vi "Calculate Formation Energies -(old).vi"(4 "N Extrinsic Atoms":i32, 5 "Fermi (electron) energy (eV)":dbl=-2.0, 6 "# Extra Electrons":i32, 7 "Reference Elemental Bulk Energies":T3={"Energy of CdTe (eV/atom)"=-2.489625, "Energy of Cd (eV/atom)"=-0.9039318, "Energy of Te (eV/atom)"=-3.1404524}, 8 "N (Te,ideal - Te,defect)":i32, 9 "N (Cd,Ideal - Cd,Defect)":i32, 10 "Reference Pure Structure Energy":dbl=-358.247, 11 "Final Total Defect Energy (eV)":dbl=-2.48963) -> (2 "Formation Energy (Te-Rich)":dbl, 3 "Formation Energy (Cd-Rich)":dbl)   [LabVIEW 2010]
panel:
  in  "System Array":T1(array[cluster])
  in  "System Cluster":T2={"Final Total Defect Energy (eV)"=-2.48963, "Reference Pure Structure Energy"=-358.247, "N (Cd,Ideal - Cd,Defect)"=0, "N (Te,ideal - Te,defect)"=0, "# Extra Electrons"=0, "Fermi (electron) energy (eV)"=-2.0}
  out "EForm 2":dbl
  out "Ed2 2":dbl
  out "Deltau 2":dbl
  out "uCd 2":dbl
  in  "uTe 2":dbl
  in  "Energy of Extrinsic X (eV/atom)":dbl
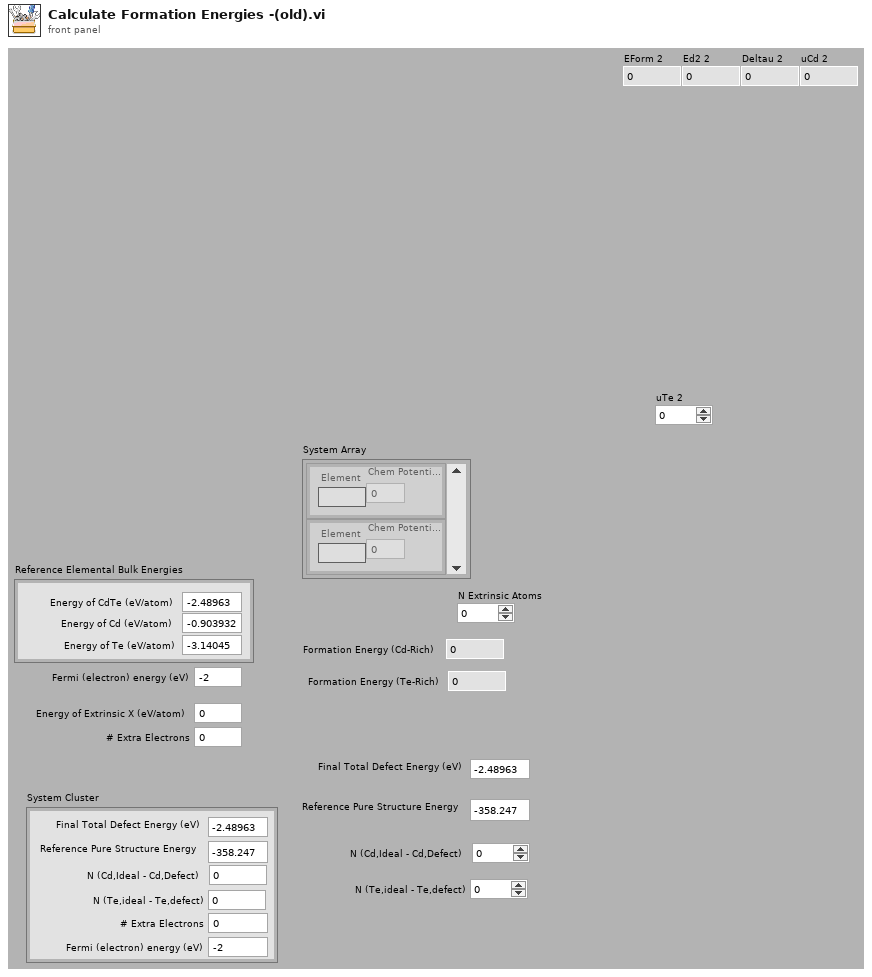
[diagram p1: front panel]
types:
  T1 = cluster{"Chem Potential (ev/atom)":dbl, "Element":string}[]
  T2 = cluster{"Final Total Defect Energy (eV)":dbl, "Reference Pure Structure Energy":dbl, "N (Cd,Ideal - Cd,Defect)":i32, "N (Te,ideal - Te,defect)":i32, "# Extra Electrons":i32, "Fermi (electron) energy (eV)":dbl}
  T3 = cluster{"Energy of CdTe (eV/atom)":dbl, "Energy of Cd (eV/atom)":dbl, "Energy of Te (eV/atom)":dbl}
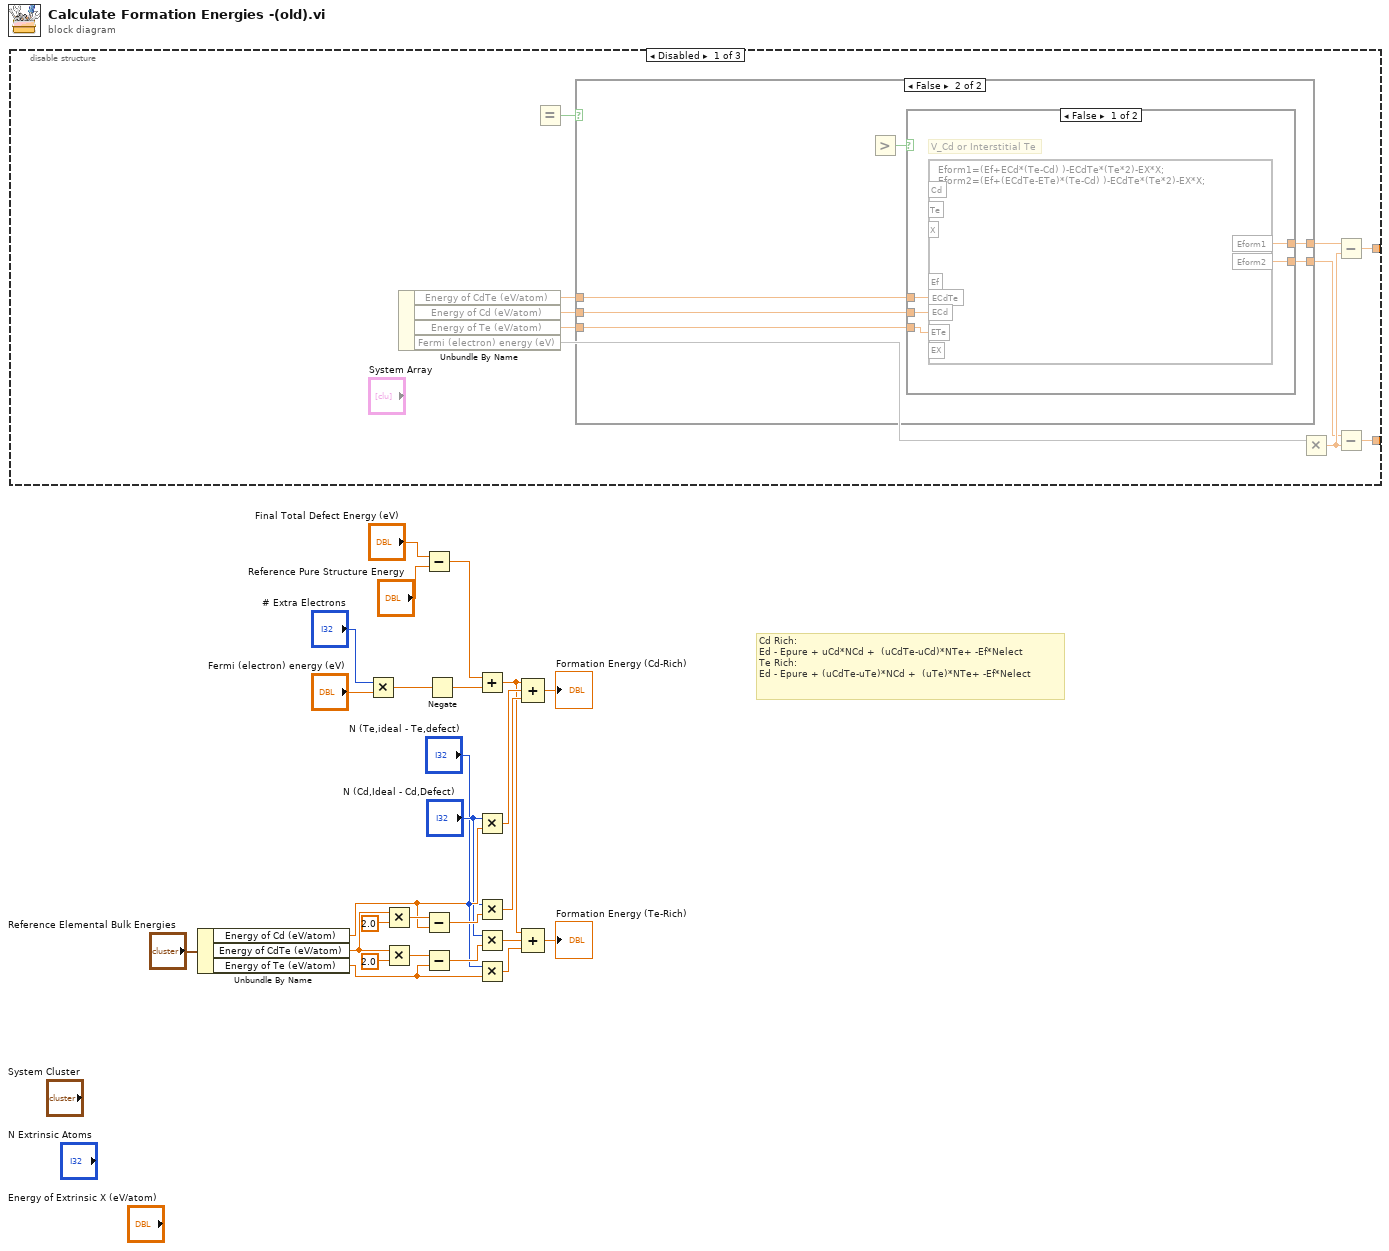
[diagram p0: block diagram]
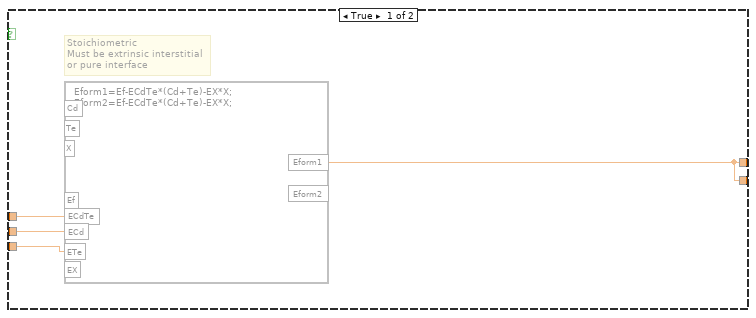
[diagram p2: hidden frame]
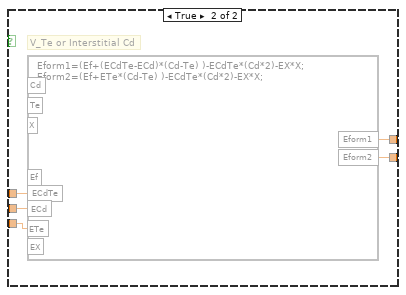
[diagram p3: hidden frame]
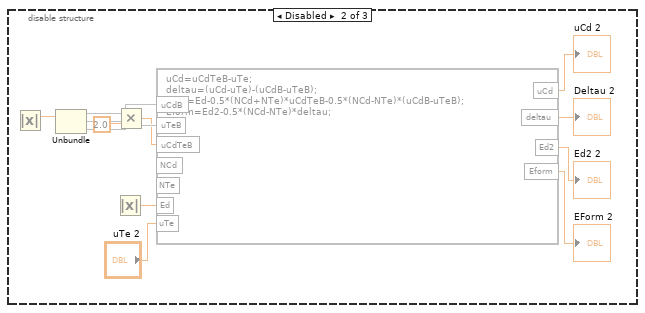
[diagram p4: hidden frame]
diagram:
  # "Cd Rich:\nEd - Epure + uCd*NCd +  (uCdTe-uCd)*NTe+ -Ef*Nelect\nTe Rich:\nEd - Epure + (uCdTe-uTe)*NCd +  (uTe)*NTe+ -Ef*Nelect"
  n1 = disable-structure shown="Disabled" {
    disable-tunnel: [w28 _ _] -> _
    disable-tunnel: [w27 _ _] -> _
    frame Disabled {
      n2 = Unbundle By Name() -> ("Energy of CdTe (eV/atom)"=w35:dbl, "Energy of Cd (eV/atom)"=w34:dbl, "Energy of Te (eV/atom)"=w33:dbl, "Fermi (electron) energy (eV)"=w32)  [unwired: 1 in]
      n3 = Equal?() -> (x = y?=w36:bool)  [unwired: 2 in]
      n4 = case shown="False" w36 {
        tunnel: w35 -> [w40 w46]
        tunnel: [w37 w42] -> w31
        tunnel: [w37 w41] -> w29
        tunnel: w34 -> [w39 w45]
        tunnel: w33 -> [w38 w44]
        frame True {
          # "Stoichiometric\nMust be extrinsic interstitial\nor pure interface"
          n5 = formula code="Eform1=Ef-ECdTe*(Cd+Te)-EX*X;\nEform2=Ef-ECdTe*(Cd+Te)-EX*X;"("ECdTe"=w40, "ECd"=w39, "ETe"=w38) -> ("Eform1"=w37:dbl)  [unwired: 5 in, 1 out]
        }
        frame False {
          n6 = Greater?() -> (0:w43:bool)  [unwired: 2 in]
          n7 = case shown="False" w43 {
            tunnel: w46 -> [w51 w56]
            tunnel: w45 -> [w50 w55]
            tunnel: w44 -> [w49 w54]
            tunnel: [w47 w52] -> w41
            tunnel: [w48 w53] -> w42
            frame False {
              # "V_Cd or Interstitial Te"
              n8 = formula code="Eform1=(Ef+ECd*(Te-Cd) )-ECdTe*(Te*2)-EX*X;\nEform2=(Ef+(ECdTe-ETe)*(Te-Cd) )-ECdTe*(Te*2)-EX*X;"("ECdTe"=w51, "ECd"=w50, "ETe"=w49) -> ("Eform1"=w48:dbl, "Eform2"=w47:dbl)  [unwired: 5 in]
            }
            frame True {
              # "V_Te or Interstitial Cd"
              n9 = formula code="Eform1=(Ef+(ECdTe-ECd)*(Cd-Te) )-ECdTe*(Cd*2)-EX*X;\nEform2=(Ef+ETe*(Cd-Te) )-ECdTe*(Cd*2)-EX*X;"("ECdTe"=w56, "ECd"=w55, "ETe"=w54) -> ("Eform1"=w53:dbl, "Eform2"=w52:dbl)  [unwired: 5 in]
            }
          }
        }
      }
      n10 = Multiply(x=w32) -> (x*y=w30:dbl)  [unwired: 1 in]
      n11 = Subtract(x=w31, y=w30) -> (x-y=w27:dbl)
      n12 = Subtract(x=w29, y=w30) -> (x-y=w28:dbl)
    }
    frame Disabled {
      n13 = Absolute Value() -> (abs(x)=w61:dbl)  [unwired: 1 in]
      n14 = Unbundle(w61) -> (w59, w68, w67)
      n15 = Absolute Value() -> (abs(x)=w60:dbl)  [unwired: 1 in]
      n16 = Multiply(x=w59, y=2.0) -> (x*y=w57:dbl)
      n17 = formula code="uCd=uCdTeB-uTe;\ndeltau=(uCd-uTe)-(uCdB-uTeB);\nEd2 =Ed-0.5*(NCd+NTe)*uCdTeB-0.5*(NCd-NTe)*(uCdB-uTeB);\nEform=Ed2-0.5*(NCd-NTe)*deltau;"("uCdB"=w68, "uTeB"=w67, "uCdTeB"=w57, "uTe"="uTe 2", "Ed"=w60) -> ("uCd"=→"uCd 2":dbl, "deltau"=→"Deltau 2":dbl, "Ed2"=→"Ed2 2":dbl, "Eform"=→"EForm 2":dbl)  [unwired: 2 in]
    }
    frame Enabled {
    }
  }
  n18 = Unbundle By Name("Reference Elemental Bulk Energies") -> ("Energy of Cd (eV/atom)"=w10:dbl, "Energy of CdTe (eV/atom)"=w11:dbl, "Energy of Te (eV/atom)"=w8:dbl)
  n19 = Multiply(x="# Extra Electrons", y="Fermi (electron) energy (eV)") -> (x*y=w5:dbl)
  n20 = Multiply(x=w11, y=2.0) -> (x*y=w12:dbl)
  n21 = Multiply(x=w11, y=2.0) -> (x*y=w16:dbl)
  n22 = Subtract(x="Final Total Defect Energy (eV)", y="Reference Pure Structure Energy") -> (x-y=w3:dbl)
  n23 = Subtract(x=w12, y=w10) -> (x-y=w9:dbl)
  n24 = Subtract(x=w16, y=w8) -> (x-y=w14:dbl)
  n25 = Negate(x=w5) -> (-x=w2:dbl)
  n26 = Add(x=w3, y=w2) -> (x+y=w1:dbl)
  n27 = Multiply(x="N (Cd,Ideal - Cd,Defect)", y=w10) -> (x*y=w20:dbl)
  n28 = Multiply(x="N (Te,ideal - Te,defect)", y=w9) -> (x*y=w18:dbl)
  n29 = Multiply(x="N (Cd,Ideal - Cd,Defect)", y=w14) -> (x*y=w19:dbl)
  n30 = Multiply(x="N (Te,ideal - Te,defect)", y=w8) -> (x*y=w17:dbl)
  n31 = Compound Arithmetic op=ADD(w1, w20, w18) -> (→"Formation Energy (Cd-Rich)":dbl)
  n32 = Compound Arithmetic op=ADD(w1, w19, w17) -> (→"Formation Energy (Te-Rich)":dbl)
